vi "命令转换.vi"(11 "启动命令":T1) -> (3 "控制命令":T2, 5 "布尔":bool)   [LabVIEW 2016, in "TimingControl.lvclass"]
uses:
  TimingControl.lvclass
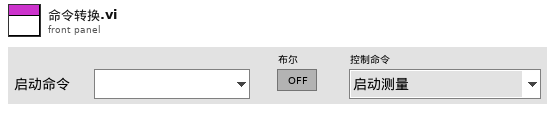
[diagram p1: front panel]
types:
  T1 = typedef "TimingControl.lvclass/启动命令选择.ctl" = enum16{"", "水样测试", "标样核查", "零点核查", "跨度核查", "空白测试", "平行样测试", "加标回收", "空白校准", "标样校准", "初始化(清洗)"}
  T2 = typedef "TimingControl.lvclass/国标控制命令.ctl" = enum16{"启动测量", "标样核查", "零点核查", "跨度核查", "空白测试", "平行样测试", "加标回收", "空白校准", "标样校准", "初始化（清洗）", "停止测试", "仪器重启", "校时", "模式设置", "测量间隔设置"}
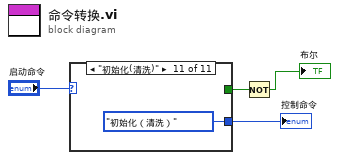
[diagram p0: block diagram]
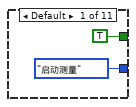
[diagram p2: hidden frame]
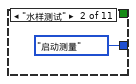
[diagram p3: hidden frame]
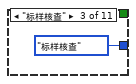
[diagram p4: hidden frame]
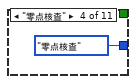
[diagram p5: hidden frame]
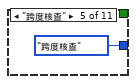
[diagram p6: hidden frame]
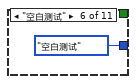
[diagram p7: hidden frame]
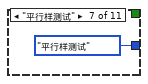
[diagram p8: hidden frame]
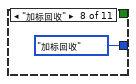
[diagram p9: hidden frame]
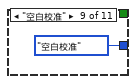
[diagram p10: hidden frame]
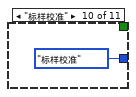
[diagram p11: hidden frame]
diagram:
  n1 = case shown="\"初始化(清洗)\"" "启动命令" {
    tunnel: [国标控制命令."启动测量" ("控制命令") 国标控制命令."启动测量" ("控制命令") 国标控制命令."标样核查" ("控制命令") 国标控制命令."零点核查" ("控制命令") 国标控制命令."跨度核查" ("控制命令") 国标控制命令."空白测试" ("控制命令") 国标控制命令."平行样测试" ("控制命令") 国标控制命令."加标回收" ("控制命令") 国标控制命令."空白校准" ("控制命令") 国标控制命令."标样校准" ("控制命令") 国标控制命令."初始化（清洗）" ("控制命令")] -> w2
    tunnel: [TRUE _ _ _ _ _ _ _ _ _ _] -> w3
    frame Default {
    }
    frame "水样测试" {
    }
    frame "标样核查" {
    }
    frame "零点核查" {
    }
    frame "跨度核查" {
    }
    frame "空白测试" {
    }
    frame "平行样测试" {
    }
    frame "加标回收" {
    }
    frame "空白校准" {
    }
    frame "标样校准" {
    }
    frame "初始化(清洗)" {
    }
  }
  "控制命令" <- w2
  n2 = Not(x=w3) -> (.not. x?=→"布尔":bool)
